vi "ADAM_DI.vi"(8 "error in":errorcluster, 10 "DUT":string) -> (0 "error in (out)":errorcluster)   [LabVIEW 2024, in "ADAM_DI.lvlib"]
doc: "This template is for the Queued Message Handler design pattern.\n\nThe Event Handling Loop generates messages based on user interface actions.\n\nThe Message Handling Loop processes messages generated by the Event Handling Loop, or by other messages. The messages are string values, so new messages can be added easily to the Message Cases case structure in the Message Handling Loop. Each message cluster can also provide an optional value for Message Data, which is a variant that can be converted to whatever message-specific data is required."
uses:
  ADAM_DI.lvlib
  support/Relay_Channel_Write.ctl
  Settings/support/Common_plc_DOs.ctl
  controls/ADAM_DI UI Data.ctl
  <vilib>/NI/Modbus Library/API/master/Modbus Master.lvclass
  PrivateControls/FGV_Queue_Control.ctl
  support/Relay_enum_IN.ctl
  595143db-fff5-4523-b6f9-8d819606822a.vi
  <vilib>/NI/Modbus Library/API/Wrapper/Create TCP Master.vi
  <vilib>/Utility/error.llb/Error Cluster From Error Code.vi
  <vilib>/ErrorRing/Error Ring.xnode
  support/Message Queue/ADAM_DI_Module Message Queue.lvlib
  support/User Event - Stop/ADAM_DI_Module User Event - Stop.lvlib
  Launcher/Launcher_DTU.lvlib
  <vilib>/NI/Modbus Library/API/Wrapper/API Main.lvlib
  Settings/Setting_Screen.lvlib
panel:
  in  "Config":string
  in  "data 2":bool[](array[boolean])
  in  "Relay_Channel_Write":T1={"Relay_CH_Array"=[{"OUTPUT_Relay_Channels"=0, "On/Off"=FALSE}, {"OUTPUT_Relay_Channels"=1, "On/Off"=FALSE}, {"OUTPUT_Relay_Channels"=2, "On/Off"=FALSE}, {"OUTPUT_Relay_Channels"=3, "On/Off"=FALSE}, {"OUTPUT_Relay_Channels"=4, "On/Off"=FALSE}, {"OUTPUT_Relay_Channels"=5, "On/Off"=FALSE}, {"OUTPUT_Relay_Channels"=6, "On/Off"=FALSE}, {"OUTPUT_Relay_Channels"=7, "On/Off"=FALSE}, {"OUTPUT_Relay_Channels"=8, "On/Off"=FALSE}, {"OUTPUT_Relay_Channels"=9, "On/Off"=FALSE}, {"OUTPUT_Relay_Channels"=10, "On/Off"=FALSE}, {"OUTPUT_Relay_Channels"=11, "On/Off"=FALSE}, {"OUTPUT_Relay_Channels"=12, "On/Off"=FALSE}, {"OUTPUT_Relay_Channels"=13, "On/Off"=FALSE}, {"OUTPUT_Relay_Channels"=14, "On/Off"=FALSE}, {"OUTPUT_Relay_Channels"=15, "On/Off"=FALSE}, {"OUTPUT_Relay_Channels"=16, "On/Off"=FALSE}, {"OUTPUT_Relay_Channels"=17, "On/Off"=FALSE}, {"OUTPUT_Relay_Channels"=18, "On/Off"=FALSE}, {"OUTPUT_Relay_Channels"=19, "On/Off"=FALSE}, {"OUTPUT_Relay_Channels"=20, "On/Off"=FALSE}, {"OUTPUT_Relay_Channels"=21, "On/Off"=FALSE}, {"OUTPUT_Relay_Channels"=22, "On/Off"=FALSE}, {"OUTPUT_Relay_Channels"=23, "On/Off"=FALSE}]} {"Relay_CH_Array"."OUTPUT_Relay_Channels" items=["CONN_SUPPLY_%d_FCT", "HB_CONN_%d_FCT", "L_IND_CONN_%d_FCT", "R_IND_CONN_%d_FCT", "SW1_%d_FCT", "SW2_%d_FCT", "CAN_H_%d_FCT", "CAN_L_%d_FCT", "CYLINDER_ON/OFF_%d_FCT", "SPARE_1_%d_FCT", "SPARE_2_%d_FCT", "Tower Red", "Tower Amber", "Tower Green", "Tower Buzzer", "SLIMRELAY_DUT_%d_FCT", "GND_DMM_%d_EOL", "CAN_H_RES_%d_EOL", "CAN_L_RES_%d_EOL", "L_IND_RES_%d_EOL", "R_IND_RES_%d_EOL", "HB_CONN_DMM_%d_EOL", "14V_RES_%d_EOL", "CAN_L_(DMM-)_%d_EOL", "CAN_H_%d_EOL", "CAN_L_%d_EOL", "14V_%d_EOL", "GND_%d_EOL", "HB_CONN_%d_EOL", "L_IND_%d_EOL", "R_IND_%d_EOL", "CYLINDER_DUT_%d_EOL", "CYL_PB_1_%d_EOL", "CYL_PB_2_%d_EOL", "DUT_PASS_%d_EOL", "DUT_FAIL_%d_EOL", "SPARE1_%d_EOL", "Tower Red_EOL", "Tower Amber_EOL", "Tower Green_EOL", "Tower Buzzer_EOL"]}
  out "discrete inputs":bool[](array[boolean])
  in  "Relay_Module_Name":string
  in  "data":bool[](array[boolean])
  out "queue name 2":string
  out "queue name":string
  out "Display <Replace Me>":string
  in  "DigitalWrite":bool
  in  "Digital Read":bool
  in  "Exit":bool
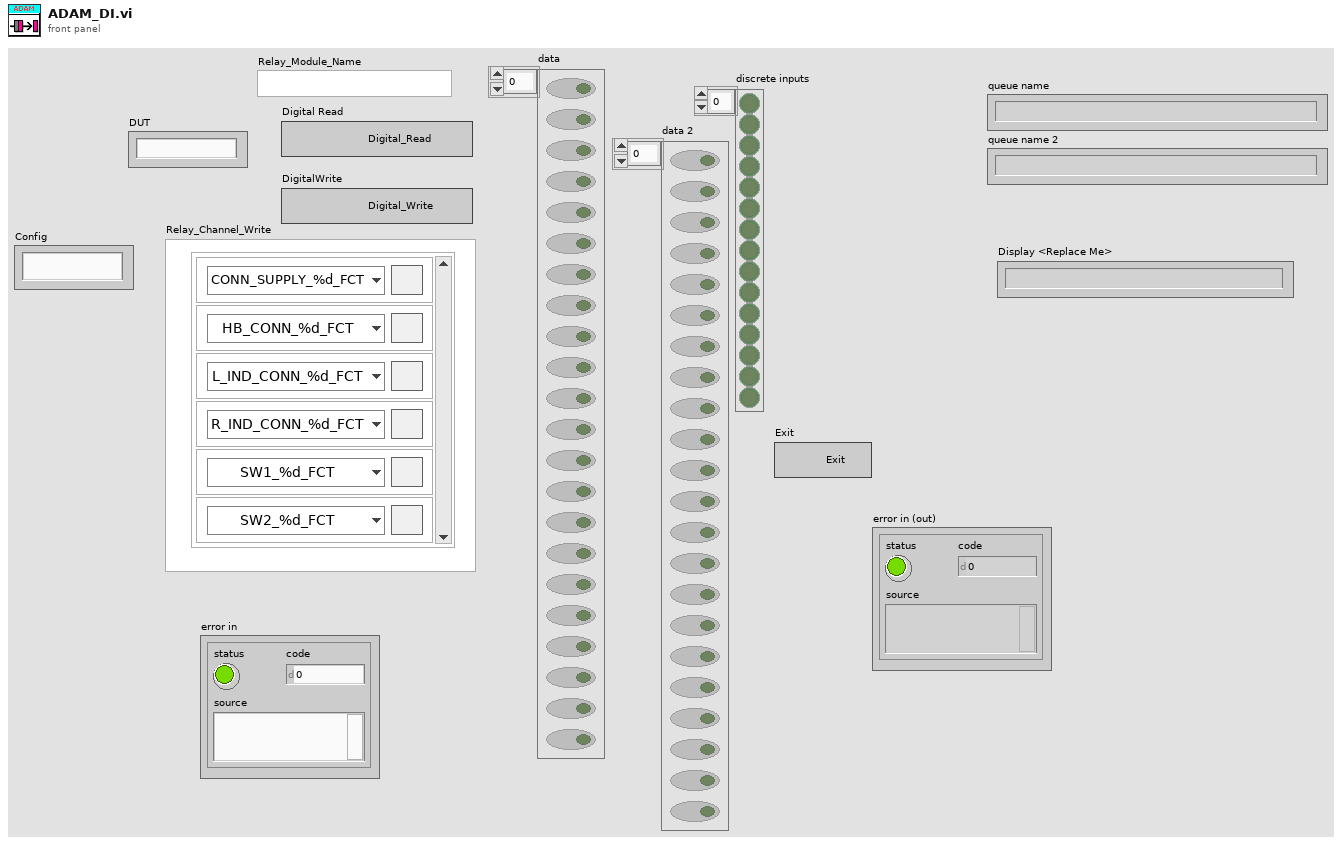
[diagram p1: front panel]
types:
  T1 = typedef "ADAM_DI.lvlib/Relay_Channel_Write.ctl" = cluster{"Relay_CH_Array":cluster{"OUTPUT_Relay_Channels":T2, "On/Off":bool}[]}
  T2 = typedef "Setting_Screen.lvlib/Common_plc_DOs.ctl" = u16
  T3 = typedef "ADAM_DI.lvlib/FGV_Queue_Control.ctl" = enum16{"Release", "Get", "Set"}
  T4 = typedef "ADAM_DI.lvlib/ADAM_DI UI Data.ctl" = cluster{"Config_Path":path, "Task_String[]":string[], "Line_String[]":string[], "DUT1_String[]":string[], "DUT2_String[]":string[], "DO_task out1":refnum<k21>, "DO_task out2":refnum<k21>, "DUT":i32, "Relay_Channel_Write":T1, "notifier out":refnum<notifier>, "serial master instance":refnum<class "Modbus Master.lvclass">, "Config":string}
  T5 = typedef "ADAM_DI.lvlib/ADAM_DI_Module Message Queue.lvlib/All Message Queues.ctl" = cluster{"UI":refnum<queue>, "QSM":refnum<queue>}
  T6 = enum16{"Read", "Write", "All_sections", "All_values", "Remove key&section"}
  T7 = cluster{"Message":string, "Message Data":variant}
  T8 = typedef "ADAM_DI.lvlib/Relay_enum_IN.ctl" = enum16{"EMERGENCY", "CONTROL ON", "START DUT 1", "START DUT 2", "STOP DUT 1", "STOP DUT 2", "PPS DUT 1", "PPS DUT 2", "REED CYL UP DUT 1", "REED CYL DOWN DUT 1", "REED CYL UP DUT 2", "REED CYL DOWN DUT 2", "LIGHT CURTAIN"}
  T9 = typedef "ADAM_DI.lvlib/Relay_Enum_OUT.ctl" = enum16{"J9 Pin_8 to Pin_1_1", "J9 Pin_8 to Pin_1_2", "J9 Pin_7 to Pin_1_1", "J9 Pin_7 to Pin_1_2", "J9 Pin_8 to Pin_7_1", "J9 Pin_8 to Pin_7_2", "J9 Pin_5 to Pin_1_1", "J9 Pin_5 to Pin_1_2", "J9 Pin_6 to Pin_1_1", "J9 Pin_6 to Pin_1_2", "J9 Pin_4 to Pin_1_1", "J9 Pin_4 to Pin_1_2", "J9 Pin_3 to Pin_1_1", "J9 Pin_3 to Pin_1_2", "PS(GND) to Pin1_1 J9", "PS(GND) to Pin1_2 J9", "PS(+14V) to Pin_3_1", "PS(+14V) to Pin_3_2", "PS(+12V) to Pin_4_1_ J9", "PS(+12V) to Pin_4_2_ J9", "PS(+12V) to Pin_5_1 J9", "PS(+12V) to Pin_5_2 J9", "PS(+12V) to Pin_6_1 J9", "PS(+12V) to Pin_6_2 J9", "Tower Amber", "Tower Red", "Tower Green", "Tower Buzzer", "PS(GND) to TP3_1", "PS(GND) to TP3_2", "PS(+14V) to TP19_1", "PS(+14V) to TP19_2", "PS(+12V) to TP33_1", "PS(+12V) to TP33_2", "PS(+12V) to TP38_1", "PS(+12V) to TP38_2", "PS(+12V) to TP40_1", "PS(+12V) to TP40_2", "TP19 (+14V) to TP3 (GND)_1", "TP19 (+14V) to TP3 (GND)_2", "TP1 (+14V) to TP3 (GND)_1", "TP1 (+14V) to TP3 (GND)_2", "TP2 (+5V) to TP3 (GND)_1", "TP2 (+5V) to TP3 (GND)_2", "TP6 (+14V) to TP9 (GND)_1", "TP6 (+14V) to TP9 (GND)_2", "TP7 (+3V8) to TP9 (GND)_1", "TP7 (+3V8) to TP9 (GND)_2", "TP11 (+14V) to TP13 (GND)_1", "TP11 (+14V) to TP13 (GND)_2", "TP12 (+3V) to TP13 (GND)_1", "TP12 (+3V) to TP13 (GND)_2", "TP5 (+3V3) to TP8 (GND)_1", "TP5 (+3V3) to TP8 (GND)_2", "TP48 (CAN_H) to TP3 (GND)_1", "TP48 (CAN_H) to TP3 (GND)_2", "TP41 (CAN_L) to TP3 (GND)_1", "TP41 (CAN_L) to TP3 (GND)_2", "TP48 (CAN_H) to TP41 (CAN_L)_1", "TP48 (CAN_H) to TP41 (CAN_L)_2", "TP38 (L_IND) to TP3 (GND)_1", "TP38 (L_IND) to TP3 (GND)_2", "TP40 (R_IND) to TP3 (GND)_1", "TP40 (R_IND) to TP3 (GND)_2", "TP33 (HB_CON) to TP3 (GND)_1", "TP33 (HB_CON) to TP3 (GND)_2", "TP19 (+14V) to TP34 (Q19-G)_1", "TP19 (+14V) to TP34 (Q19-G)_2", "TP55 (SW1) to TP3 (GND)_1", "TP55 (SW1) to TP3 (GND)_2", "TP56 (SW2) to TP3 (GND)_1", "TP56 (SW2) to TP3 (GND)_2", "TP66 WRT TP3 (GND)_1", "TP66 WRT TP3 (GND)_2", "TP19 WRT TP3_1", "TP19 WRT TP3_2", "TP1 WRT TP3_1", "TP1 WRT TP3_2", "TP2 WRT TP3_1", "TP2 WRT TP3_2", "TP7 WRT TP9_1", "TP7 WRT TP9_2", "TP12 WRT TP13_1", "TP12 WRT TP13_2", "TP5 WRT TP8_1", "TP5 WRT TP8_2", "TP22 WRT TP3_1", "TP22 WRT TP3_2", "TP52 WRT TP3(GND)_1", "TP52 WRT TP3(GND)_2", "TP50 WRT TP3(GND)_1", "TP50 WRT TP3(GND)_2", "TP51 WRT TP3(GND)_1", "TP51 WRT TP3(GND)_2"}
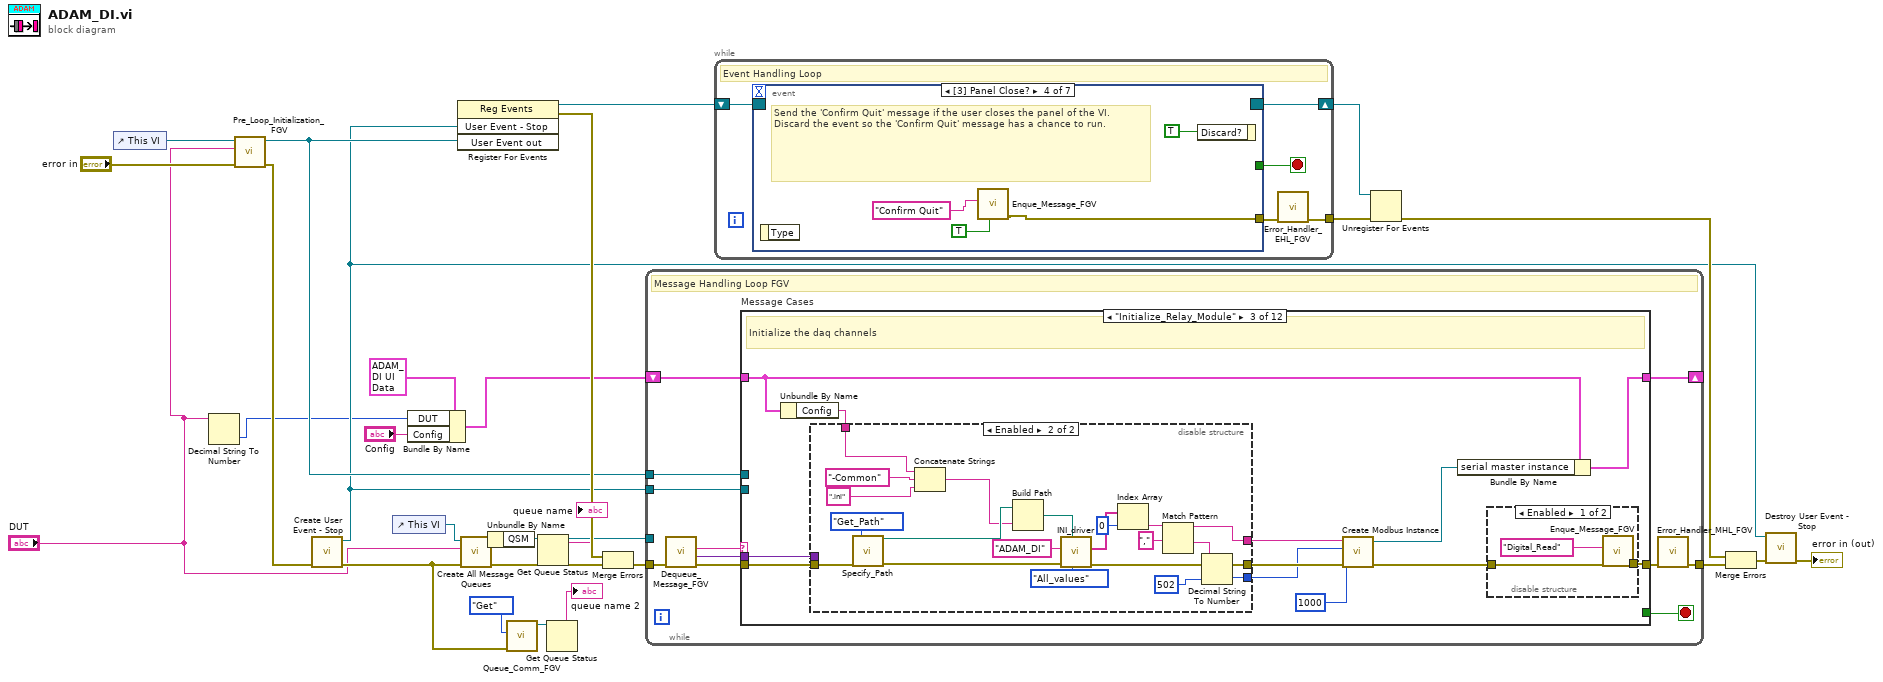
[diagram p0: block diagram]
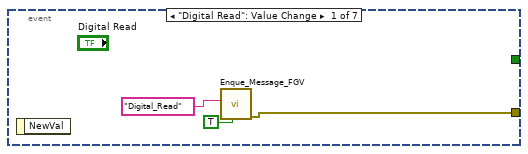
[diagram p2: hidden frame]
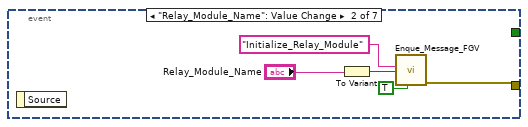
[diagram p3: hidden frame]
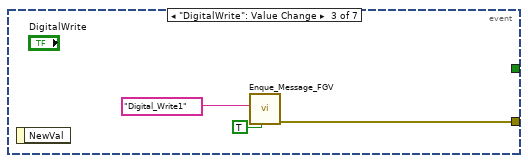
[diagram p4: hidden frame]
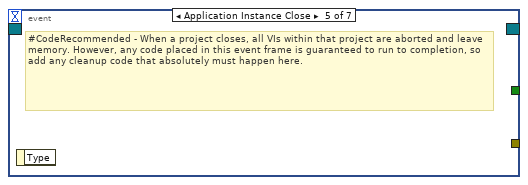
[diagram p5: hidden frame]
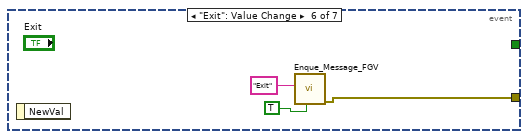
[diagram p6: hidden frame]
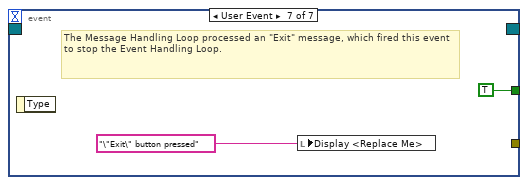
[diagram p7: hidden frame]
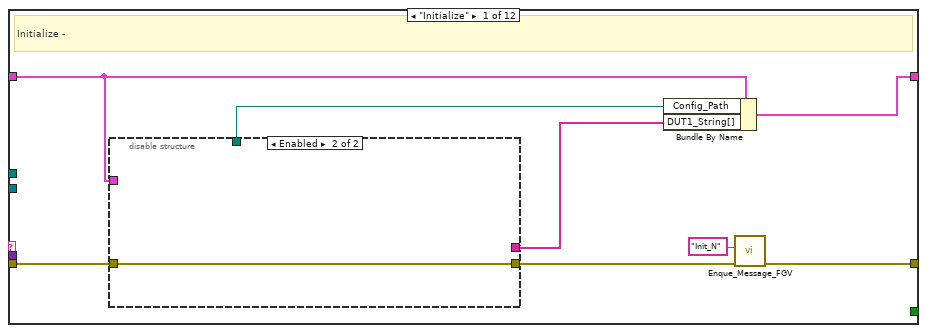
[diagram p8: hidden frame]
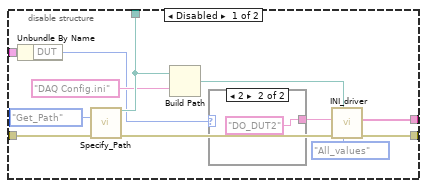
[diagram p9: hidden frame]
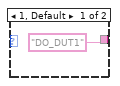
[diagram p10: hidden frame]
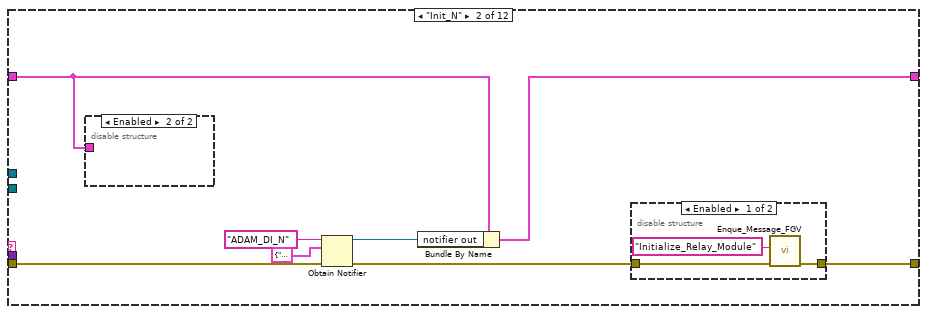
[diagram p11: hidden frame]
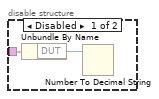
[diagram p12: hidden frame]
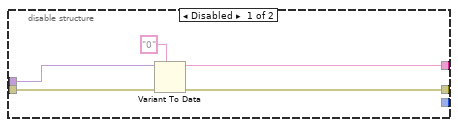
[diagram p15: hidden frame]
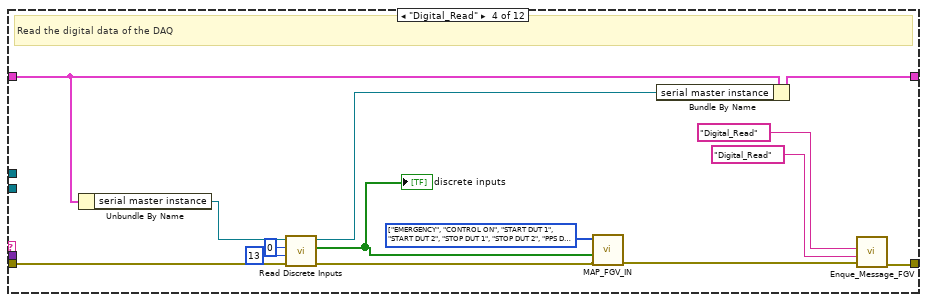
[diagram p16: hidden frame]
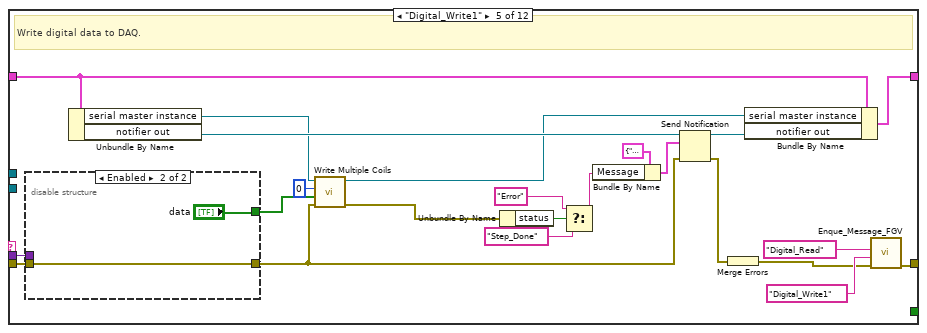
[diagram p17: hidden frame]
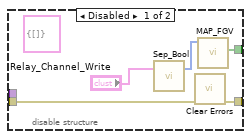
[diagram p18: hidden frame]
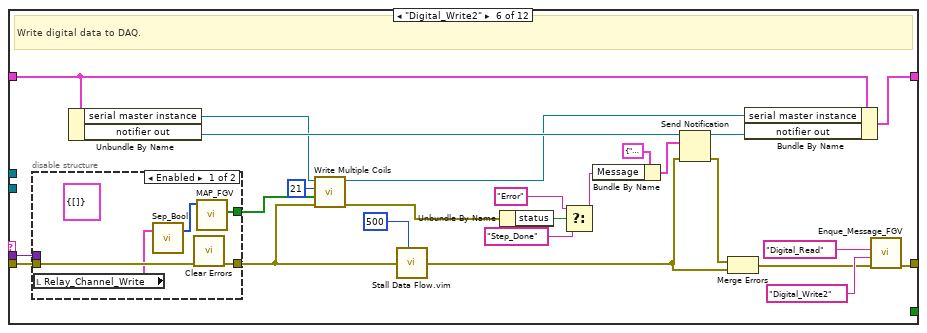
[diagram p19: hidden frame]
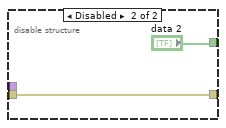
[diagram p20: hidden frame]
diagram:
  n1 = control-ref of="This VI"() -> (w17:refnum<vi>)
  n2 = Decimal String To Number(string="DUT") -> (number=w1:i32)  [unwired: 2 in, 1 out]
  n3 = call "Pre_Loop_Initialization_FGV.vi"("error in (no error)"="error in", "DUT"="DUT", "VI in"=w17) -> ("error out"=w15:errorcluster, "User Event out"=w6:refnum<user-event>)  [unwired: 7 in]
  n4 = call "Create User Event - Stop.vi"("error in (no error)"=w15) -> ("error out"=w10:errorcluster, "User Event - Stop"=w5:refnum<user-event>)  [unwired: 9 in]
  n5 = control-ref of="This VI"() -> (w13:refnum<vi>)
  n6 = Bundle By Name(cluster=T4 {"Config_Path"=path "", "Task_String[]"=[], "Line_String[]"=[], "DUT1_String[]"=[], "DUT2_String[]"=[], "DO_task out1"="", "DO_task out2"="", "DUT"=0, "Relay_Channel_Write"={"Relay_CH_Array"=[]}, "notifier out"=refnum, "serial master instance"=refnum, "Config"=""} ("Data Cluster"), "DUT"=w1, "Config"="Config") -> (w4:T4)
  n7 = register-events(w5, w6) -> (reference out=w20:refnum<event-registration>, error out=w18:errorcluster)  [unwired: 2 in]
  n8 = call "Create All Message Queues.vi"("error in (no error)"=w10, "DUT"="DUT", "This VI"=w13) -> ("error out"=w29:errorcluster, "Message Queues out"=w28:T5)  [unwired: 7 in]
  n9 = Unbundle By Name(w28) -> ("QSM"=w26:refnum<queue>)
  n10 = call "Queue_Comm_FGV.vi"("error in (no error)"=w10, "Enum"=FGV_Queue_Control."Get") -> ("queue Out"=w8:refnum<queue>)  [unwired: 8 in, 1 out]
  n11 = Get Queue Status(queue=w26) -> (queue out=w12:refnum<queue>, queue name=→"queue name":string)  [unwired: 2 in, 6 out]
  n12 = Get Queue Status(queue=w8) -> (queue name=→"queue name 2":string)  [unwired: 2 in, 7 out]
  n13 = Merge Errors(w18, w29) -> (w19:errorcluster)
  n14 = while {
    tunnel: w12 -> [_]
    shift-right: [w39] -> _
    shift-left: w4 -> [w40]
    tunnel: w6 -> [w37]
    tunnel: w19 -> [w36]
    tunnel: [w31] -> w27
    tunnel: w5 -> [w30]
    stop <- w38 stop-if-true
    # "Message Handling Loop FGV"
    n15 = call "Dequeue_Message_FGV.vi"("error in (no error)"=w36) -> ("error out"=w35:errorcluster, "Message Data"=w34:variant, "Message"=w33:string)  [unwired: 8 in]
    n16 = case "Message Cases" shown="\"Initialize_Relay_Module\"" w33 {
      selector: w33 -> [_ _ _ _ _ _ _ _ _ _ _ w247]
      tunnel: w35 -> [w47 w71 w87 w128 w151 w183 w206 w215 w225 w228 w237 _]
      tunnel: [w48 w64 w89 w130 w155 w187 w210 w216 w219 w230 w232 w248] -> w32
      tunnel: w40 -> [w42 w70 w79 w129 w152 w184 w207 w217 w224 w231 w238 w249]
      tunnel: [w45 w67 w83 w124 w150 w182 w205 w217 w224 w231 w238 w249] -> w39
      tunnel: [_ _ _ _ _ _ _ _ _ _ TRUE _] -> w38
      tunnel: w34 -> [_ _ w85 _ w148 w180 _ w214 w223 _ _ _]
      tunnel: w37 -> [_ _ _ _ _ _ _ _ _ _ w244 _]
      tunnel: w30 -> [_ _ _ _ _ _ _ _ _ _ w241 _]
      frame "Initialize" {
        # "Initialize -"
        n17 = disable-structure shown="Enabled" {
          disable-tunnel: w47 -> [w60 w63]
          disable-tunnel: [w57 w63] -> w44
          disable-tunnel: [w56 _] -> w43
          disable-tunnel: w42 -> [w52 _]
          disable-tunnel: [w50 _] -> w41
          frame Disabled {
            n18 = Unbundle By Name(w52) -> ("DUT"=w49:i32)
            n19 = call "Specify_Path.vi"("Path_Enum"=enum16{"Find_Path", "Get_Path"}."Get_Path", "error in (no error)"=w60) -> ("Configurations"=w56:path, "error out"=w59:errorcluster)  [unwired: 6 in, 6 out]
            n20 = Build Path(base path=w56, name or relative path="DAQ Config.ini") -> (appended path=w54:path)
            n21 = case shown="2" w49 {
              tunnel: ["DO_DUT1" ("String") "DO_DUT2" ("String")] -> w51
              frame 1, Default {
              }
              frame 2 {
              }
            }
            n22 = call "INI_driver.vi"("Enum"=T6."All_values", "instrument file path"=w54, "error in (no error)"=w59, "Section"=w51) -> ("error out"=w57:errorcluster, "Values out"=w50:string[])  [unwired: 4 in, 2 out]
          }
          frame Enabled {
          }
        }
        n23 = Bundle By Name(cluster=w42, "Config_Path"=w43, "DUT1_String[]"=w41) -> (w45:T4)
        n24 = call "Enque_Message_FGV.vi"("error in (no error)"=w44, "Message"="Init_N") -> ("error out"=w48:errorcluster)  [unwired: 9 in]
      }
      frame "Init_N" {
        n25 = disable-structure shown="Enabled" {
          disable-tunnel: w70 -> [w73 _]
          frame Disabled {
            n26 = Unbundle By Name(w73) -> ("DUT"=w72:i32)
            n27 = Number To Decimal String(number=w72) -> ()  [unwired: 1 in, 1 out]
          }
          frame Enabled {
          }
        }
        n28 = Obtain Notifier(name (unnamed)="ADAM_DI_N" ("String"), notification data type=T7 {"Message"="", "Message Data"=variant} ("notification"), error in (no error)=w71) -> (notifier out=w66:refnum<notifier>, error out=w65:errorcluster)  [unwired: 1 in, 1 out]
        n29 = Bundle By Name(cluster=w70, "notifier out"=w66) -> (w67:T4)
        n30 = disable-structure shown="Enabled" {
          disable-tunnel: w65 -> [w75 w77]
          disable-tunnel: [w74 w77] -> w64
          frame Enabled {
            n31 = call "Enque_Message_FGV.vi"("error in (no error)"=w75, "Message"="Initialize_Relay_Module") -> ("error out"=w74:errorcluster)  [unwired: 9 in]
          }
          frame Disabled {
          }
        }
      }
      frame "Initialize_Relay_Module" {
        # "Initialize the daq channels"
        n32 = Unbundle By Name(w79) -> ("Config"=w78:string)
        n33 = disable-structure shown="Enabled" {
          disable-tunnel: w87 -> [w98 w111]
          disable-tunnel: [w97 w110] -> w86
          disable-tunnel: w85 -> [w96 _]
          disable-tunnel: [w95 w103] -> w84
          disable-tunnel: [_ w100] -> w81
          disable-tunnel: w78 -> [_ w99]
          frame Disabled {
            n34 = Variant To Data(error in=w98, type="0", Variant=w96) -> (data=w95:string, error out=w97:errorcluster)
          }
          frame Enabled {
            n35 = call "Specify_Path.vi"("Path_Enum"=enum16{"Find_Path", "Get_Path"}."Get_Path", "error in (no error)"=w111) -> ("Configurations"=w117:path, "error out"=w114:errorcluster)  [unwired: 6 in, 6 out]
            n36 = Concatenate Strings(w99, "-Common" ("string"), ".ini" ("string")) -> (w107:string)
            n37 = Build Path(base path=w117, name or relative path=w107) -> (appended path=w116:path)
            n38 = call "INI_driver.vi"("Enum"=T6."All_values", "instrument file path"=w116, "error in (no error)"=w114, "Section"="ADAM_DI") -> ("error out"=w110:errorcluster, "Values out"=w112:string[])  [unwired: 4 in, 2 out]
            n39 = Index Array(array=w112, index=0) -> (element=w105:string)
            n40 = Match Pattern(string=w105, regular expression=",") -> (before substring=w103:string, after substring=w102:string)  [unwired: 1 in, 2 out]
            n41 = Decimal String To Number(string=w102, default (0L)=u16 502 ("port (502)")) -> (number=w100:u16)  [unwired: 1 in, 1 out]
          }
        }
        n42 = call-poly <vilib>:"Create Modbus Instance.vi"("error in"=w86, "connect timeout ms"=1000, "port (502)"=w81, "address"=w84) -> ("error out"=w88:errorcluster, "TCP master instance"=w82:refnum<class "Modbus Master.lvclass">)  [unwired: 6 in]
        n43 = Bundle By Name(cluster=w79, "serial master instance"=w82) -> (w83:T4)
        n44 = disable-structure shown="Enabled" {
          disable-tunnel: [w92 w93] -> w89
          disable-tunnel: w88 -> [w90 w93]
          frame Enabled {
            n45 = call "Enque_Message_FGV.vi"("error in (no error)"=w90, "Message"="Digital_Read") -> ("error out"=w92:errorcluster)  [unwired: 9 in]
          }
          frame Disabled {
          }
        }
      }
      frame "Digital_Read" {
        w122 = T8[] [enum."EMERGENCY", enum."CONTROL ON", enum."START DUT 1", enum."START DUT 2", enum."STOP DUT 1", enum."STOP DUT 2", enum."PPS DUT 1", enum."PPS DUT 2", enum."REED CYL UP DUT 1", enum."REED CYL DOWN DUT 1", enum."REED CYL UP DUT 2", enum."REED CYL DOWN DUT 2", enum."LIGHT CURTAIN"] items=["EMERGENCY", "CONTROL ON", "START DUT 1", "START DUT 2", "STOP DUT 1", "STOP DUT 2", "PPS DUT 1", "PPS DUT 2", "REED CYL UP DUT 1", "REED CYL DOWN DUT 1", "REED CYL UP DUT 2", "REED CYL DOWN DUT 2", "LIGHT CURTAIN"] ("PLC_BOOL_IN")
        # "Read the digital data of the DAQ"
        n46 = Unbundle By Name(w129) -> ("serial master instance"=w127:refnum<class "Modbus Master.lvclass">)
        n47 = call-dynamic "Read Discrete Inputs.vi"("error in"=w128, "number of inputs"=u16 13, "starting address"=u16 0, "Modbus master in"=w127) -> ("error out"=w121:errorcluster, "discrete inputs"=w119:bool[], "Modbus master out"=w123:refnum<class "Modbus Master.lvclass">)  [unwired: 5 in]
        "discrete inputs" <- w119
        n48 = call "MAP_FGV_IN.vi"("error in (no error)"=w121, "DOs"=w119, "Relay_ENUM_IN"=w122) -> ("error out"=w120:errorcluster)  [unwired: 6 in, 2 out]
        n49 = Bundle By Name(cluster=w129, "serial master instance"=w123) -> (w124:T4)
        n50 = call "Enque_Message_FGV.vi"("error in (no error)"=w120, "Message Data"="Digital_Read" ("\"Do Something\" button pressed"), "Message"="Digital_Read") -> ("error out"=w130:errorcluster)  [unwired: 8 in]
      }
      frame "Digital_Write1" {
        # "Write digital data to DAQ."
        n51 = disable-structure shown="Enabled" {
          disable-tunnel: w151 -> [w160 w162]
          disable-tunnel: w148 -> [_ _]
          disable-tunnel: [w158 w162] -> w139
          disable-tunnel: [w157 "data"] -> w133
          frame Disabled {
            (unwired) T1 {"Relay_CH_Array"=[]} ("DAQ_Write")
            n52 = call "Sep_Bool.vi"("Relay_Channel_Write"="Relay_Channel_Write") -> ("DO_Enum"=w159:T9[])  [unwired: 1 in, 1 out]
            n53 = call <vilib>:"Clear Errors.vi"("error in (no error)"=w160) -> ("error out"=w158:errorcluster)  [unwired: 5 in, 1 out]
            n54 = call "MAP_FGV.vi"("Relay_Channel_Out"=w159) -> ("DOs_out"=w157:bool[])  [unwired: 8 in, 2 out]
          }
          frame Enabled {
          }
        }
        n55 = Unbundle By Name(w152) -> ("serial master instance"=w136:refnum<class "Modbus Master.lvclass">, "notifier out"=w147:refnum<notifier>)
        n56 = call-dynamic "Write Multiple Coils.vi"("error in"=w139, "coils to write"=w133, "starting address"=u16 0, "Modbus master in"=w136) -> ("error out"=w137:errorcluster, "Modbus master out"=w135:refnum<class "Modbus Master.lvclass">)  [unwired: 6 in]
        n57 = Unbundle By Name(w137) -> ("status"=w145:bool)
        n58 = Select(t="Error", s=w145, f="Step_Done") -> (s? t:f=w143:string)
        n59 = Bundle By Name(cluster=T7 {"Message"="", "Message Data"=variant} ("notification"), "Message"=w143) -> (w142:T7)
        n60 = Send Notification(notification=w142, notifier=w147, error in (no error)=w139) -> (notifier out=w138:refnum<notifier>, error out=w140:errorcluster)
        n61 = Merge Errors(w140) -> (w149:errorcluster)
        n62 = Bundle By Name(cluster=w152, "serial master instance"=w135, "notifier out"=w138) -> (w150:T4)
        n63 = call "Enque_Message_FGV.vi"("error in (no error)"=w149, "Message Data"="Digital_Write1" ("\"Do Something Else\" button pressed"), "Message"="Digital_Read") -> ("error out"=w155:errorcluster)  [unwired: 8 in]
      }
      frame "Digital_Write2" {
        # "Write digital data to DAQ."
        n64 = disable-structure shown="Enabled" {
          disable-tunnel: w183 -> [w192 w194]
          disable-tunnel: w180 -> [_ _]
          disable-tunnel: [w190 w194] -> w171
          disable-tunnel: [w189 "data 2"] -> w163
          frame Enabled {
            (unwired) T1 {"Relay_CH_Array"=[]} ("DAQ_Write")
            n65 = local read "Relay_Channel_Write"() -> (w188:T1)
            n66 = call "Sep_Bool.vi"("Relay_Channel_Write"=w188) -> ("DO_Enum"=w191:T9[])  [unwired: 1 in, 1 out]
            n67 = call <vilib>:"Clear Errors.vi"("error in (no error)"=w192) -> ("error out"=w190:errorcluster)  [unwired: 5 in, 1 out]
            n68 = call "MAP_FGV.vi"("Relay_Channel_Out"=w191) -> ("DOs_out"=w189:bool[])  [unwired: 8 in, 2 out]
          }
          frame Disabled {
          }
        }
        n69 = Unbundle By Name(w184) -> ("serial master instance"=w166:refnum<class "Modbus Master.lvclass">, "notifier out"=w179:refnum<notifier>)
        n70 = call-dynamic "Write Multiple Coils.vi"("error in"=w171, "coils to write"=w163, "starting address"=u16 21, "Modbus master in"=w166) -> ("error out"=w167:errorcluster, "Modbus master out"=w165:refnum<class "Modbus Master.lvclass">)  [unwired: 6 in]
        n71 = call "Stall Data Flow.vim"("value in"=w171, "milliseconds to wait"=u32 500) -> ("value out"=w169:errorcluster)  [unwired: 1 out]
        n72 = Unbundle By Name(w167) -> ("status"=w177:bool)
        n73 = Select(t="Error", s=w177, f="Step_Done") -> (s? t:f=w175:string)
        n74 = Bundle By Name(cluster=T7 {"Message"="", "Message Data"=variant} ("notification"), "Message"=w175) -> (w174:T7)
        n75 = Send Notification(notification=w174, notifier=w179, error in (no error)=w169) -> (notifier out=w170:refnum<notifier>, error out=w172:errorcluster)
        n76 = Merge Errors(w172, w169) -> (w181:errorcluster)
        n77 = Bundle By Name(cluster=w184, "serial master instance"=w165, "notifier out"=w170) -> (w182:T4)
        n78 = call "Enque_Message_FGV.vi"("error in (no error)"=w181, "Message Data"="Digital_Write2" ("\"Do Something Else\" button pressed"), "Message"="Digital_Read") -> ("error out"=w187:errorcluster)  [unwired: 8 in]
      }
      frame "Towerlamp" {
        (unwired) T1 {"Relay_CH_Array"=[]} ("DAQ_Write")
        # "Write digital data to DAQ."
        n79 = local read "Relay_Channel_Write"() -> (w196:T1)
        n80 = Unbundle By Name(w207) -> ("serial master instance"=w201:refnum<class "Modbus Master.lvclass">, "notifier out"=w203:refnum<notifier>)
        n81 = call "Sep_Bool.vi"("Relay_Channel_Write"=w196) -> ("DO_Enum"=w197:T9[])  [unwired: 1 in, 1 out]
        n82 = call <vilib>:"Clear Errors.vi"("error in (no error)"=w206) -> ("error out"=w202:errorcluster)  [unwired: 5 in, 1 out]
        n83 = call "MAP_FGV.vi"("Relay_Channel_Out"=w197) -> ("DOs_out"=w198:bool[])  [unwired: 8 in, 2 out]
        n84 = call-dynamic "Write Multiple Coils.vi"("error in"=w202, "coils to write"=w198, "starting address"=u16 21, "Modbus master in"=w201) -> ("error out"=w195:errorcluster, "Modbus master out"=w200:refnum<class "Modbus Master.lvclass">)  [unwired: 6 in]
        n85 = Merge Errors(w195) -> (w204:errorcluster)
        n86 = Bundle By Name(cluster=w207, "serial master instance"=w200, "notifier out"=w203) -> (w205:T4)
        n87 = call "Enque_Message_FGV.vi"("error in (no error)"=w204, "Message Data"="Tower lamp" ("\"Do Something Else\" button pressed"), "Message"="Digital_Read") -> ("error out"=w210:errorcluster)  [unwired: 8 in]
      }
      frame "Update Display" {
        # "Update Display - Convert the message data to a string to display in the Data Display indicator."
        n88 = Variant To Data(error in=w215, type="", Variant=w214) -> (data=→"Display <Replace Me>":string, error out=w212:errorcluster)
        n89 = Merge Errors(w212) -> (w216:errorcluster)
      }
      frame "Error" {
        # "Error - Display an error dialog. This message is sent by the \"Error Handler\" VIs at the end of other loops in this application."
        n90 = Variant To Data(error in=w225, type=errorcluster {"status"=FALSE, "code"=0, "source"=""} ("error constant"), Variant=w223) -> (data=w221:errorcluster, error out=w220:errorcluster)
        n91 = call <vilib>:"Simple Error Handler.vi"("error in (no error)"=w221) -> ()  [unwired: 4 in, 5 out]
        n92 = call <vilib>:"Clear Errors.vi"("error in (no error)"=w220) -> ("error out"=w218:errorcluster)  [unwired: 5 in, 1 out]
        n93 = Merge Errors(w218) -> (w219:errorcluster)
      }
      frame "Confirm Quit" {
        # "#CodeNeeded - If you want to provide an \"Are you sure\" dialog (or some other notification) before the application exits, place that code here. This message is typically sent from a Panel Close? event."
        # "Confirm Quit - Message that can confirm whether or not the user wants to exit the application."
        n94 = call "Enque_Message_FGV.vi"("Priority"=TRUE ("Priority Message? (F)"), "error in (no error)"=w228, "Message"="Exit") -> ("error out"=w229:errorcluster)  [unwired: 8 in]
        n95 = Merge Errors(w229) -> (w230:errorcluster)
      }
      frame "Exit" {
        # "Exit - Exit the application."
        n96 = Unbundle By Name(w238) -> ("serial master instance"=w233:refnum<class "Modbus Master.lvclass">, "notifier out"=w235:refnum<notifier>)
        n97 = call "Queue_Comm_FGV.vi"("error in (no error)"=w237, "Enum"=FGV_Queue_Control."Release") -> ("error Out"=w242:errorcluster)  [unwired: 8 in, 1 out]
        n98 = call-dynamic "Shutdown.vi"("error in"=w237, "Modbus master in"=w233) -> ("error out"=w234:errorcluster)  [unwired: 9 in]
        n99 = Release Notifier(notifier=w235, error in (no error)=w237) -> (error out=w236:errorcluster)  [unwired: 1 in, 2 out]
        n100 = call "Fire User Event - Stop.vi"("User Event - Stop"=w241) -> ("error out"=w239:errorcluster)  [unwired: 10 in]
        n101 = call "Fire User Event - Stop.vi"("User Event - Stop"=w244) -> ("error out"=w240:errorcluster)  [unwired: 10 in]
        n102 = Merge Errors(w234, w236, w240, w239, w242) -> (w245:errorcluster)
        n103 = call <vilib>:"Clear Errors.vi"("error in (no error)"=w245) -> ("error out"=w232:errorcluster)  [unwired: 5 in, 1 out]
      }
      frame Default {
        # "'Default' case only runs if there is a message that isn't defined in any of the other cases.  Output a programming error."
        n104 = xnode "Error Ring"("parameter 0"=w247) -> ("error out"=w248:errorcluster)
      }
    }
    n105 = call "Error_Handler_MHL_FGV.vi"("error in (no error)"=w32) -> ("error Out"=w31:errorcluster)  [unwired: 10 in]
  }
  n106 = while {
    shift-right: [w260] -> w23
    shift-left: w20 -> [w261]
    tunnel: [w257] -> w21
    stop <- w259 stop-if-true
    # "Event Handling Loop"
    n107 = event shown="[3] Panel Close?" {
      selector: w261 -> [_ _ _ _ _ _ _]
      dyn-events: [_ _ _ _ _ _ _] -> w260
      timeout: _ -> [_ _ _ _ _ _ _]
      tunnel: [_ _ _ _ _ _ TRUE ("Discard?")] -> w259
      tunnel: [w263 w267 w270 w275 _ w279 _] -> w258
      event "Digital Read": Value Change {
        n108 = event-data() -> ()  [unwired: 1 in, 1 out]
        n109 = call "Enque_Message_FGV.vi"("Priority"=TRUE ("Priority Message? (F)"), "Message"="Digital_Read") -> ("error out"=w263:errorcluster)  [unwired: 9 in]
      }
      event "Relay_Module_Name": Value Change {
        n110 = event-data() -> ()  [unwired: 1 in, 1 out]
        n111 = To Variant(anything="Relay_Module_Name") -> (Variant=w266:variant)
        n112 = call "Enque_Message_FGV.vi"("Priority"=TRUE ("Priority Message? (F)"), "Message Data"=w266, "Message"="Initialize_Relay_Module") -> ("error out"=w267:errorcluster)  [unwired: 8 in]
      }
      event "DigitalWrite": Value Change {
        n113 = event-data() -> ()  [unwired: 1 in, 1 out]
        n114 = call "Enque_Message_FGV.vi"("Priority"=TRUE ("Priority Message? (F)"), "Message"="Digital_Write1") -> ("error out"=w270:errorcluster)  [unwired: 9 in]
      }
      event Panel Close? {
        # "Send the 'Confirm Quit' message if the user closes the panel of the VI. Discard the event so the 'Confirm Quit' message has a chance to run."
        n115 = event-data() -> ()  [unwired: 1 in, 1 out]
        n116 = call "Enque_Message_FGV.vi"("Priority"=TRUE ("Priority Message? (F)"), "Message"="Confirm Quit") -> ("error out"=w275:errorcluster)  [unwired: 9 in]
        n117 = event-data("Discard?"=TRUE) -> ()  [unwired: 1 in, 1 out]
      }
      event Application Instance Close {
        # "#CodeRecommended - When a project closes, all VIs within that project are aborted and leave memory. However, any code placed in this event frame is guaranteed to run to completion, so add any cleanup code that absolutely must happen here."
        n118 = event-data() -> ()  [unwired: 1 in, 1 out]
      }
      event "Exit": Value Change {
        n119 = event-data() -> ()  [unwired: 1 in, 1 out]
        n120 = call "Enque_Message_FGV.vi"("Priority"=TRUE ("Priority Message? (F)"), "Message"="Exit") -> ("error out"=w279:errorcluster)  [unwired: 9 in]
      }
      event User Event {
        # "The Message Handling Loop processed an \"Exit\" message, which fired this event to stop the Event Handling Loop."
        n121 = event-data() -> ()  [unwired: 1 in, 1 out]
        n122 = local write "Display <Replace Me>"("\"Exit\" button pressed" ("VI Stopped")) -> ()
      }
    }
    n123 = call "Error_Handler_EHL_FGV.vi"("error in (no error)"=w258) -> ("error Out"=w257:errorcluster)  [unwired: 10 in]
  }
  n124 = Unregister For Events(event registration refnum=w23, error in=w21) -> (error out=w24:errorcluster)
  n125 = Merge Errors(w24, w27) -> (w25:errorcluster)
  n126 = call "Destroy User Event - Stop.vi"("error in (no error)"=w25, "User Event - Stop"=w5) -> ("error out"=→"error in (out)":errorcluster)  [unwired: 9 in]
